vi "ScreenShot.vi"() -> ()   [LabVIEW 2014]
panel:
  out "error out":errorcluster
  in  "error in (no error)":errorcluster
  in  "Access Path":path
  # "Note : remember to add the file format behind the file name"
  # "Ex : test.jpg"
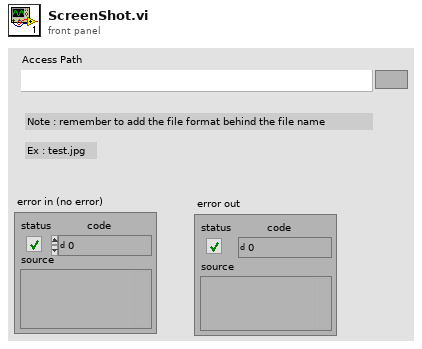
[diagram p1: front panel]
types:
  T1 = typedef "imagedata.ctl" = cluster{"image type":i32, "image depth":i32, "image":u8[], "mask":u8[], "colors":u32[], "Rectangle":cluster{"left":i16, "top":i16, "right":i16, "bottom":i16}}
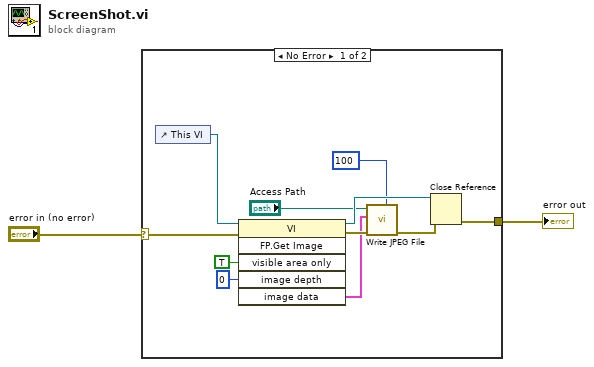
[diagram p0: block diagram]
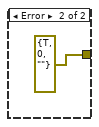
[diagram p2: hidden frame]
diagram:
  n1 = case shown="No Error" "error in (no error)" {
    selector: "error in (no error)" -> [w3 _]
    tunnel: [w13 errorcluster {"status"=TRUE, "code"=0, "source"=""} ("error out")] -> w1
    frame No Error {
      n2 = control-ref of="This VI"() -> (w10:refnum<vi>)
      n3 = invoke class="VI" method="FP.Get Image"(reference=w10, error in=w3, "visible area only"=TRUE ("Visible Area Only"), "image depth"=0 ("Image Depth")) -> (reference out=w9:refnum<vi>, error out=w11:errorcluster, "image data"=w7:T1)  [unwired: 2 in, 3 out]
      n4 = call <vilib>:"Write JPEG File.vi"("quality (80)"=100, "error in (no error)"=w11, "image data"=w7, "path to JPEG file"="Access Path") -> ("error out"=w12:errorcluster)  [unwired: 6 in, 1 out]
      n5 = Close Reference(reference=w9, error in (no error)=w12) -> (error out=w13:errorcluster)
    }
    frame Error {
    }
  }
  "error out" <- w1
